vi "Do.vi"(8 "error in (no error)":errorcluster, 10 "Actor in":refnum<class "Actor.lvclass">, 11 "Acquired data result msg":refnum<class "Acquired data result msg.lvclass">) -> (0 "error out":errorcluster, 2 "Actor out":refnum<class "Actor.lvclass">)   [LabVIEW 2015, in "Acquired data result msg.lvclass"]
doc: "(<B>Filename</B>: Actor Framework.lvlib:Message.lvclass:Do.vi)\n\nDefines what a message does when it is received by an actor. Generally, a message instructs an actor to invoke one of its methods. By default, this method does nothing. A child class must override it to define behavior. Create a child class by using the Actor Framework Message Maker dialog box."
uses:
  Acquire data request message/Acquired data result msg.lvclass
  <vilib>/ActorFramework/Actor/Actor.lvclass
  Gage digitizer actor.lvclass
  Acquire data request message/Acquired data result msg.lvclass/Acquired data result msg.ctl
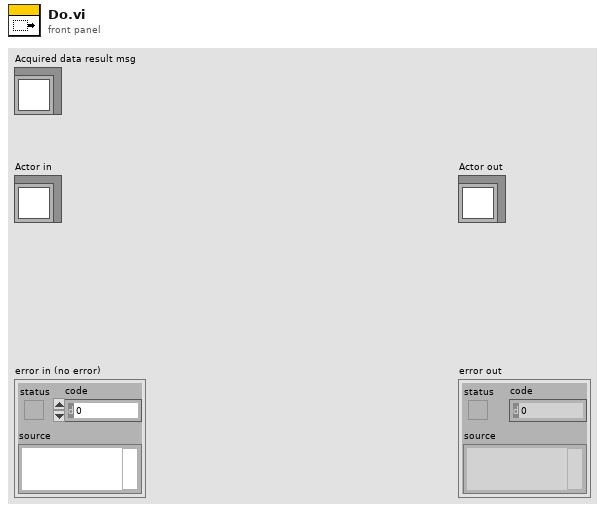
[diagram p1: front panel]
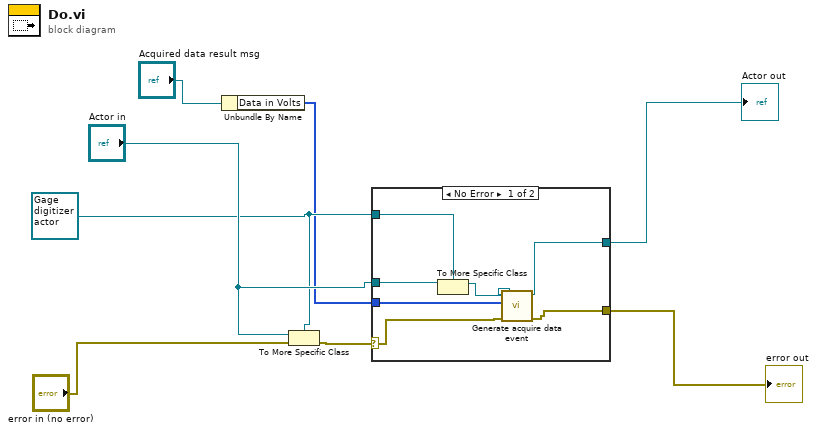
[diagram p0: block diagram]
diagram:
  w3 = refnum<class "Gage digitizer actor.lvclass"> refnum ("Gage digitizer actor.lvclass")
  n1 = Unbundle By Name("Acquired data result msg") -> ("Data in Volts"=w1:i16[])
  n2 = To More Specific Class(target class=w3, reference="Actor in", error in="error in (no error)") -> (error out=w8:errorcluster)  [unwired: 1 out]
  n3 = case shown="No Error" w8 {
    selector: w8 -> [w11 w17]
    tunnel: "Actor in" -> [w15 w16]
    tunnel: [w10 w17] -> w5
    tunnel: w3 -> [w14 _]
    tunnel: [w12 w16] -> w4
    tunnel: w1 -> [w9 _]
    frame No Error {
      n4 = To More Specific Class(target class=w14, reference=w15) -> (specific class reference=w13:refnum<class "Gage digitizer actor.lvclass">)  [unwired: 1 in, 1 out]
      n5 = call-dynamic "Generate acquire data event.vi"("error in (no error)"=w11, "Data in Volts"=w9, "Gage digitizer actor in"=w13) -> ("error out"=w10:errorcluster, "Gage digitizer actor out"=w12:refnum<class "Gage digitizer actor.lvclass">)  [unwired: 7 in]
    }
    frame Error {
    }
  }
  "error out" <- w5
  "Actor out" <- w4
